vi "test_get_testimages.vi"() -> ()   [LabVIEW 2018, in "LV-0mq-Julia_roundtrip-lib.lvlib"]
uses:
  LV-0mq-Julia_roundtrip-lib.lvlib
  Commands.ctl
  Server or client state.ctl
  18e075e7-4cd2-4762-b22d-c93500a3c2e5.vi
  b3d2dca1-5e2b-4c2b-a3b1-37e7c47fa7d2.vi
  StackFrame.ctl
  detailed error info.ctl
panel:
  out "img_type":string
  out "picture":picture
  out "detailed error info 2":T1
  in  "select image":u16(ring) items=["autumn_leaves.png", "blobs.gif", "cameraman.tif", "chelsea.png", "coffee.png", "earth_apollo17.jpg", "fabio_color_256.png", "fabio_color_512.png", "fabio_gray_256.png", "fabio_gray_512.png", "hela-cells.tif", "house.tif", "jetplane.tif", "lake_color.tif", "lake_gray.tif", "lena_color_256.tif", "lena_color_512.tif", "lena_gray_256.tif", "lena_gray_512.tif", "lena_gray_16bit.png", "livingroom.tif", "lighthouse.png", "mandril_color.tif", "mandril_gray.tif", "mandrill.tiff", "m51.tif", "moonsurface.tiff", "mountainstream.png", "peppers_color.tif", "peppers_gray.tif", "pirate.tif", "resolution_test_512.tif", "resolution_test_1920.tif", "toucan.png", "walkbridge.tif", "woman_blonde.tif", "woman_darkhair.tif"]
  in  "Start Server from LabVIEW":bool=TRUE
  in  "next":bool
  in  "stop LV only":bool
  in  "stop":bool
  out "detailed error info":T1
  out "Jl Server state out":T3
  out "final error":errorcluster
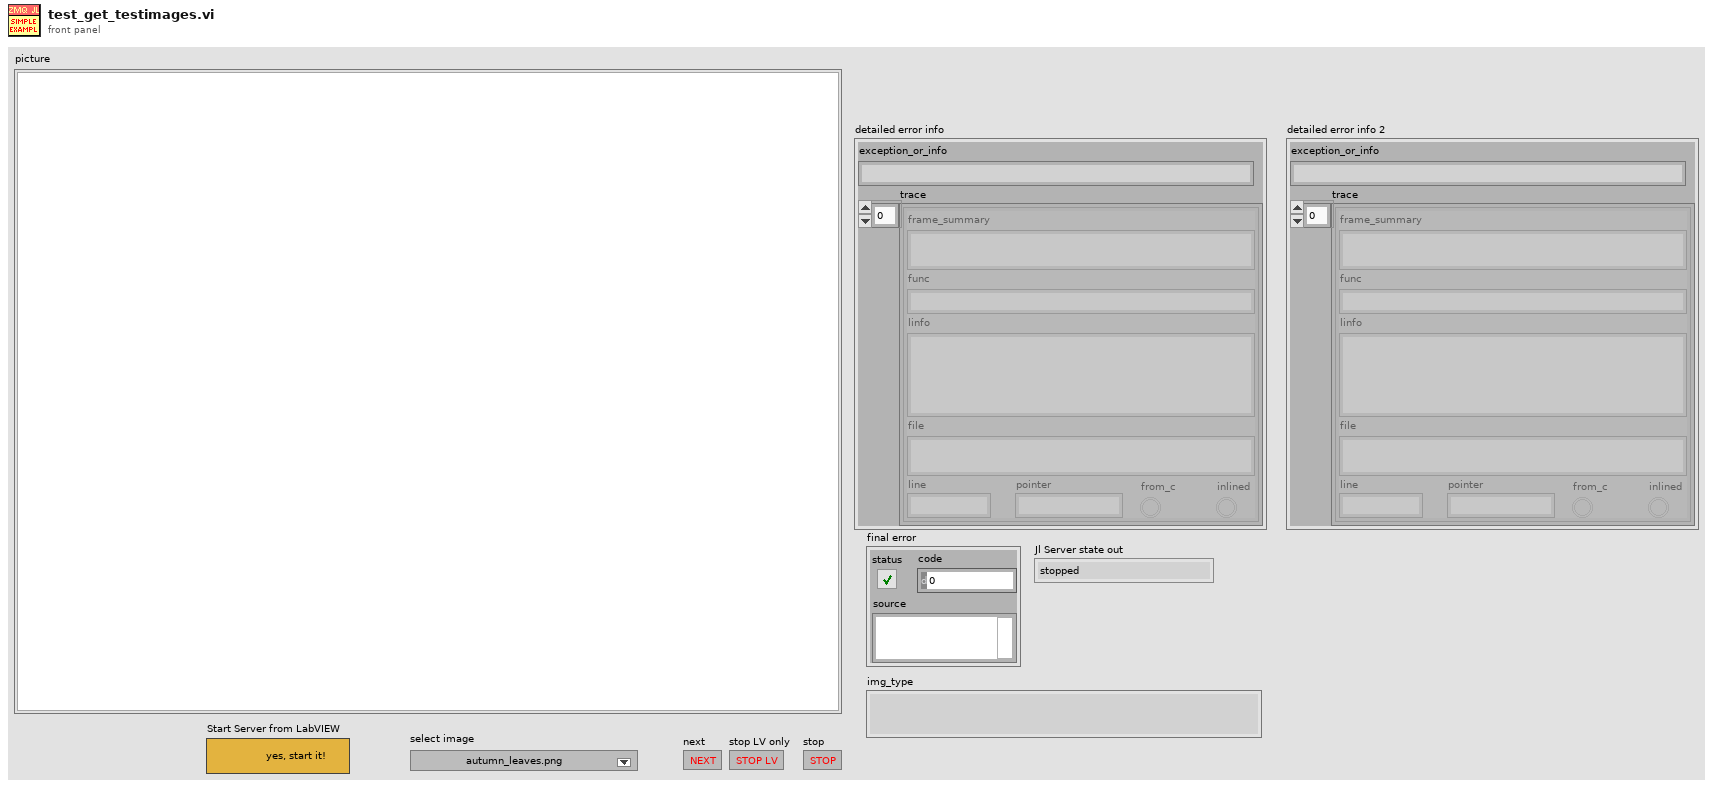
[diagram p1: front panel]
types:
  T1 = typedef "LV-0mq-Julia_roundtrip-lib.lvlib/detailed error info.ctl" = cluster{"exception_or_info":string, "trace":T2[]}
  T2 = typedef "LV-0mq-Julia_roundtrip-lib.lvlib/StackFrame.ctl" = cluster{"frame_summary":string, "func":string, "linfo":string, "file":string, "line":i32, "pointer":u64, "from_c":bool, "inlined":bool}
  T3 = typedef "LV-0mq-Julia_roundtrip-lib.lvlib/Server or client state.ctl" = enum16{"stopped", "running", "unknown"}
  T4 = typedef "LV-0mq-Julia_roundtrip-lib.lvlib/Commands.ctl" = enum16{"Start Jl-server & Init LV-client", "Send request & Get response ", "Stop Jl-server & Cleanup LV-client", "Cleanup LV-client", "Start Jl-server", "Stop Jl-server", "Init LV-Client", "Cleanup LV-Client", "(not allowed)", "Set LV Client state", "Set Jl Server state", "set ZMQ timeout", "read ZMQ timeout", "read-out state"}
  T5 = typedef "imagedata.ctl" = cluster{"image type":i32, "image depth":i32, "image":u8[], "mask":u8[], "colors":u32[], "Rectangle":cluster{"left":i16, "top":i16, "right":i16, "bottom":i16}}
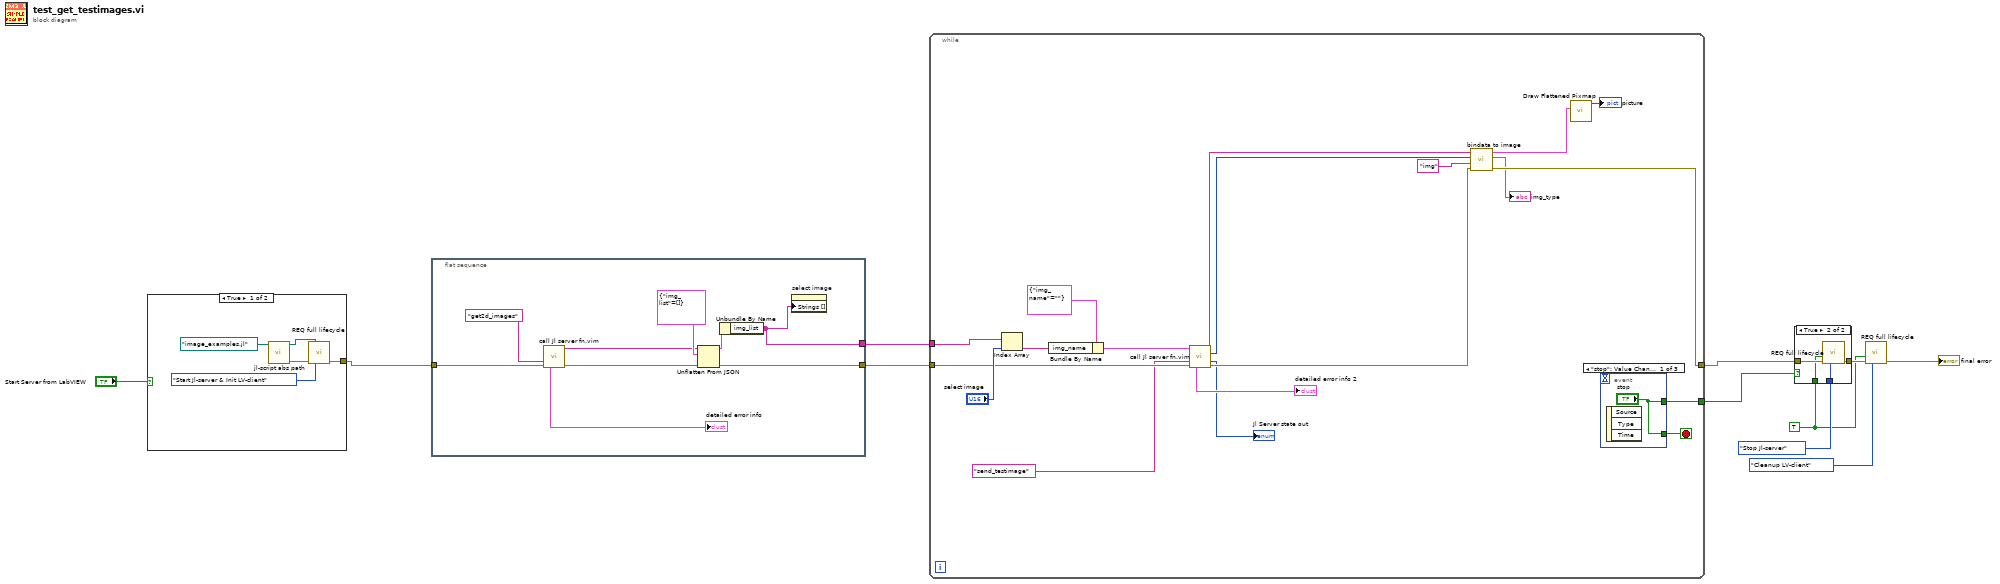
[diagram p0: block diagram]
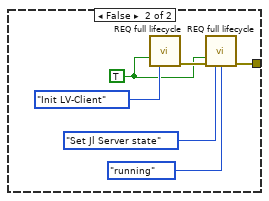
[diagram p2: hidden frame]
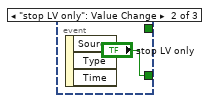
[diagram p3: hidden frame]
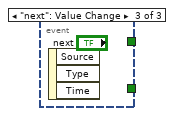
[diagram p4: hidden frame]
diagram:
  w7 = TRUE ("Force command")
  n1 = case shown="True" "Start Server from LabVIEW" {
    tunnel: [w15 w17] -> w4
    frame True {
      n2 = call "jl-script abs path.vi"("Julia user functions script"=path "image_examples.jl") -> ("error out"=w12:errorcluster, "script abs path"=w13:path)  [unwired: 9 in]
      n3 = call "REQ full lifecycle.vi"("Julia user functions script"=w13, "error in"=w12, "command"=Commands."Start Jl-server & Init LV-client") -> ("error out"=w15:errorcluster)  [unwired: 6 in, 6 out]
    }
    frame False {
      w19 = TRUE ("Force command")
      n4 = call "REQ full lifecycle.vi"("Force command"=w19, "command"=Commands."Init LV-Client") -> ("error out"=w21:errorcluster)  [unwired: 7 in, 6 out]
      n5 = call "REQ full lifecycle.vi"("Force command"=w19, "error in"=w21, "command"=Commands."Set Jl Server state", "Jl Server state in"=Server_or_client_state."running") -> ("error out"=w17:errorcluster)  [unwired: 5 in, 6 out]
    }
  }
  n6 = flat-sequence {
    tunnel: [w31] -> w3
    tunnel: w4 -> [w26]
    tunnel: [w28] -> w1
    frame #0 {
      n7 = call "call Jl server fn.vim"("fun2call"="get2d_images", "error in (no error)"=w26) -> ("JSON received"=w25:string, "detailed error info"=→"detailed error info":T1, "error out"=w24:errorcluster)  [unwired: 7 in, 4 out]
      n8 = Unflatten From JSON(JSON string=w25, type and defaults=cluster{"img_list":string[]} {"img_list"=[]} ("parsed response"), error in (no error)=w24) -> (value=w29:cluster{"img_list":string[]}, error out=w31:errorcluster)  [unwired: 4 in]
      n9 = Unbundle By Name(w29) -> ("img_list"=w28:string[])
      n10 = property on="select image" class="Ring (strict)"("Strings []"=w28) -> ()  [unwired: 2 in, 2 out]
    }
  }
  n11 = while {
    tunnel: [w49] -> w6
    tunnel: w3 -> [w39]
    tunnel: [w44] -> w2
    tunnel: w1 -> [w48]
    stop <- w50 stop-if-true
    n12 = Index Array(array=w48, index="select image") -> (element=w45:string)
    n13 = Bundle By Name(cluster=cluster{"img_name":string} {"img_name"=""} ("parsed response"), "img_name"=w45) -> (w37:cluster{"img_name":string})
    n14 = call "call Jl server fn.vim"("Arguments 1"=w37, "fun2call"="send_testimage", "error in (no error)"=w39) -> ("JSON received"=w35:string, "binary data received"=w36:u8[], "Jl Server state out"=→"Jl Server state out":T3, "detailed error info"=→"detailed error info 2":T1, "error out"=w40:errorcluster)  [unwired: 6 in, 2 out]
    n15 = call "bindata to image.vi"("error in (no error)"=w40, "name"="img", "binary data in"=w36, "JSON in"=w35) -> ("error out"=w44:errorcluster, 2:→"img_type", "img out"=w42:T5)  [unwired: 5 in]
    n16 = call <vilib>:"Draw Flattened Pixmap.vi"("image data"=w42) -> ("new picture"=→"picture":picture)  [unwired: 8 in]
    n17 = event shown="[0] \"stop\": Value Change" {
      selector: _ -> [_ _ _]
      dyn-events: _ -> [_ _ _]
      timeout: _ -> [_ _ _]
      tunnel: ["stop" "stop LV only" _] -> w50
      tunnel: ["stop" _ _] -> w49
      event "stop": Value Change {
        n18 = event-data() -> ()  [unwired: 1 in, 3 out]
      }
      event "stop LV only": Value Change {
        n19 = event-data() -> ()  [unwired: 1 in, 3 out]
      }
      event "next": Value Change {
        n20 = event-data() -> ()  [unwired: 1 in, 3 out]
      }
    }
  }
  n21 = case shown="True" w6 {
    tunnel: w2 -> [w53 w57]
    tunnel: Commands."Stop Jl-server" ("command") -> [_ w56]
    tunnel: [w53 w55] -> w10
    tunnel: w7 -> [_ w54]
    frame False {
    }
    frame True {
      n22 = call "REQ full lifecycle.vi"("Force command"=w54, "error in"=w57, "command"=w56) -> ("error out"=w55:errorcluster)  [unwired: 6 in, 6 out]
    }
  }
  n23 = call "REQ full lifecycle.vi"("Force command"=w7, "error in"=w10, "command"=Commands."Cleanup LV-client") -> ("error out"=→"final error":errorcluster)  [unwired: 6 in, 6 out]
